vi "Read Transfer Names.vi"(8 "error in (no error)":errorcluster, 11 "dsf refnum":T1) -> (0 "error out":errorcluster, 1 "names":string[](array[string]), 3 "dsf refnum out":T1)   [LabVIEW 2017, in "DSF Configuration API.lvlib"]
doc: "Gets the names of all sections from the configuration data identified by <B>dsf refnum</B>."
uses:
  DSF Configuration API.lvlib
  Controls/DSF Config Data RefNum.ctl
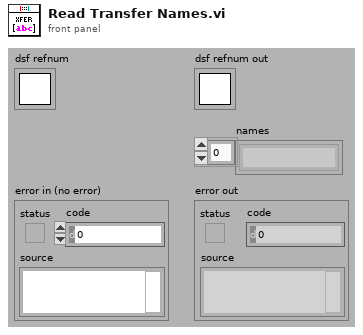
[diagram p1: front panel]
types:
  T1 = typedef "DSF Configuration API.lvlib/DSF Config Data RefNum.ctl" = refnum<k1>
  T2 = typedef "DSF Configuration API.lvlib/DSF Configuration Reference.ctl" = refnum<data-value>
  T3 = typedef "DSF Configuration API.lvlib/Config Data.ctl" = cluster{"dsf configuration":T4, "path":path, "dirty":bool}
  T4 = typedef "DSF Configuration API.lvlib/DSF Config.ctl" = cluster{"dsfversion":T5, "version":T5, "plugins":T6[], "groups":T9[], "transfers":T11[], "channels":T13[], "settings":T15[]}
  T5 = typedef "DSF Configuration API.lvlib/Version Info.ctl" = cluster{"major":u32, "minor":u32, "fix":u32, "build":string}
  T6 = typedef "DSF Configuration API.lvlib/DSF Plugin.ctl" = cluster{"id":string, "values":T7}
  T7 = typedef "DSF Configuration API.lvlib/DSF Plugin Info.ctl" = cluster{"type":string, "timing":T8, "group ids":string[], "settings id":string}
  T8 = typedef "DSF Configuration API.lvlib/DSF Timing Info.ctl" = cluster{"priority":i32, "decimation":i32, "offset":i32}
  T9 = typedef "DSF Configuration API.lvlib/DSF Group.ctl" = cluster{"id":string, "values":T10}
  T10 = typedef "DSF Configuration API.lvlib/DSF Group Info.ctl" = cluster{"direction":i32, "timing":T8, "transfer ids":string[], "settings id":string}
  T11 = typedef "DSF Configuration API.lvlib/DSF Transfer.ctl" = cluster{"id":string, "values":T12}
  T12 = typedef "DSF Configuration API.lvlib/DSF Transfer Info.ctl" = cluster{"byte order":i32, "channel ids":string[], "settings id":string}
  T13 = typedef "DSF Configuration API.lvlib/DSF Channel.ctl" = cluster{"id":string, "values":T14}
  T14 = typedef "DSF Configuration API.lvlib/DSF Channel Info.ctl" = cluster{"count":i32, "offset":i32, "data type":i32, "resource path":string, "settings id":string}
  T15 = typedef "DSF Configuration API.lvlib/DSF Settings.ctl" = cluster{"id":string, "values":T16}
  T16 = typedef "DSF Configuration API.lvlib/DSF Settings Info.ctl" = cluster{"key":string, "value":string}[]
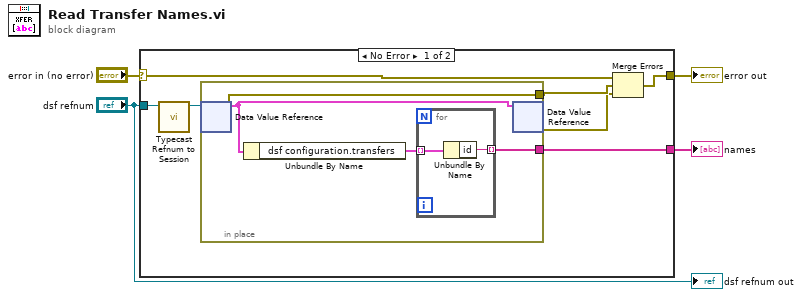
[diagram p0: block diagram]
diagram:
  n1 = case shown="No Error" "error in (no error)" {
    selector: "error in (no error)" -> [w9 w18]
    tunnel: [w11 _] -> w2
    tunnel: [w7 w18] -> w3
    tunnel: "dsf refnum" -> [w10 _]
    frame No Error {
      n2 = call "Typecast Refnum to Session.vi"("dsf refnum in"=w10) -> ("DSF Configuration Reference out"=w8:T2)  [unwired: 10 in]
      n3 = in-place {
        in-place-border: [w15] -> w11
        in-place-border: [w12] -> w6
        n4 = in-place-dvr #1(w8) -> (w13:T3, w12:errorcluster)
        n5 = Unbundle By Name(w13) -> ("dsf configuration.transfers"=w14:T11[])
        n6 = for {
          tunnel: w14 -> [w16] mode=indexing
          tunnel: [w17] -> w15 mode=indexing
          n7 = Unbundle By Name(w16) -> ("id"=w17:string)
        }
        n8 = in-place-dvr #1(w13) -> (w5:errorcluster)  [unwired: 1 out]
      }
      n9 = Merge Errors(w9, w6, w5) -> (w7:errorcluster)
    }
    frame Error {
    }
  }
  "error out" <- w3
  "names" <- w2
  "dsf refnum out" <- "dsf refnum"
